vi "HB_ReadAI.vi"   [LabVIEW 2016]
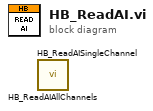
[diagram p0: block diagram]
diagram:
  n1 = call <vilib>:"HB_ReadAIAllChannels.vi"() -> ()  [unwired: 8 in, 4 out]
  n2 = call <vilib>:"HB_ReadAISingleChannel.vi"() -> ()  [unwired: 8 in, 4 out]
